vi "GetType.vi"(8 "error in (no error)":errorcluster, 11 "Create Channel Arbitrary Waveform [ACH] Msg in":refnum<class "Create Channel Arbitrary Waveform [ACH] Msg.lvclass">) -> (0 "error out":errorcluster, 2 "Data Sample":variant, 3 "Create Channel Arbitrary Waveform [ACH] Msg out":refnum<class "Create Channel Arbitrary Waveform [ACH] Msg.lvclass">)   [LabVIEW 2014, in "CS++Fgen.lvlib" / "Create Channel Arbitrary Waveform [ACH] Msg.lvclass"]
doc: "This VI delivers a sample of the data type format the message expects."
uses:
  Create Channel Arbitrary Waveform [ACH] Msg.lvclass
  Create Channel Arbitrary Waveform [ACH] Msg.lvclass/Create Channel Arbitrary Waveform [ACH] Msg.ctl
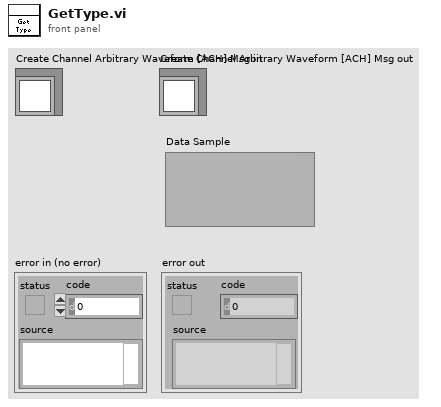
[diagram p1: front panel]
types:
  T1 = cluster{"waveform data array (empty)":dbl[], "Channel Name (\"\")":string}
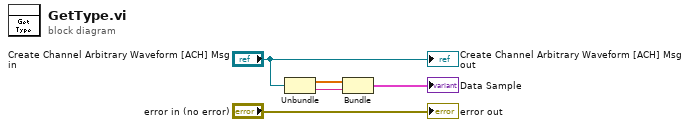
[diagram p0: block diagram]
diagram:
  n1 = Unbundle("Create Channel Arbitrary Waveform [ACH] Msg in") -> (w3:dbl[], w2:string)
  n2 = Bundle("waveform data array (empty)"=w3, "Channel Name (\"\")"=w2) -> (→"Data Sample":T1)  [unwired: 1 in]
  "error out" <- "error in (no error)"
  "Create Channel Arbitrary Waveform [ACH] Msg out" <- "Create Channel Arbitrary Waveform [ACH] Msg in"
